vi "Calculate Texture Gradient.vi"(10 "P2":T2 {"v" min=0 max=1 step=0.1; "u" min=0 max=1 step=0.1}, 11 "P1":T2 {"v" min=0 max=1 step=0.1; "u" min=0 max=1 step=0.1}) -> (3 "Line Parameters":T1)   [LabVIEW 2022 SP3, in "Raster.lvlib"]
uses:
  UV.ctl
  Line Parameters.ctl
  Raster.lvlib
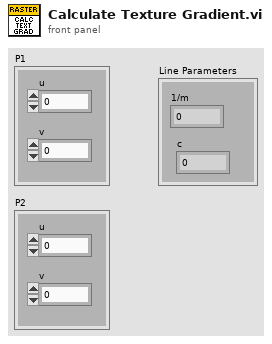
[diagram p1: front panel]
types:
  T1 = typedef "Raster.lvlib/Line Parameters.ctl" = cluster{"1/m":sgl, "c":sgl}
  T2 = typedef "Raster.lvlib/UV.ctl" = cluster{"u":sgl, "v":sgl}
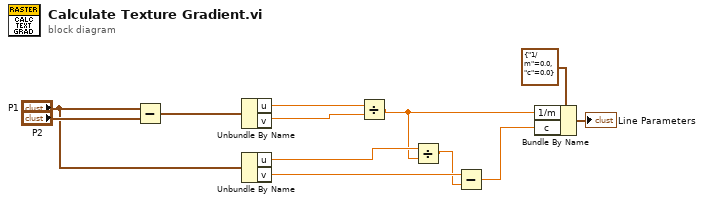
[diagram p0: block diagram]
diagram:
  n1 = Subtract(x="P1", y="P2") -> (x-y=w11:T2)
  n2 = Unbundle By Name(w11) -> ("u"=w10:sgl, "v"=w9:sgl)
  n3 = Unbundle By Name("P1") -> ("u"=w6:sgl, "v"=w7:sgl)
  n4 = Divide(x=w10, y=w9) -> (x/y=w2:sgl)
  n5 = Divide(x=w6, y=w2) -> (x/y=w5:sgl)
  n6 = Subtract(x=w7, y=w5) -> (x-y=w3:sgl)
  n7 = Bundle By Name(cluster=T1 {"1/m"=0.0, "c"=0.0} ("Line"), "1/m"=w2, "c"=w3) -> (→"Line Parameters":T1)
